vi "cubic and deadbands subvi.vi"(8 "Axis2":dbl, 9 "Axis1":dbl) -> (2 "Axis2":dbl, 3 "Axis1":dbl)   [LabVIEW 2017]
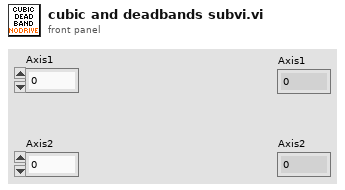
[diagram p1: front panel]
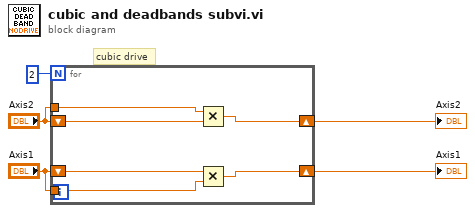
[diagram p0: block diagram]
diagram:
  # "cubic drive"
  n1 = for {
    N: 2 -> [_]
    shift-right: [w6] -> w3
    shift-left: "Axis1" -> [w11]
    shift-right: [w7] -> w4
    shift-left: "Axis2" -> [w9]
    tunnel: "Axis1" -> [w10]
    tunnel: "Axis2" -> [w8]
    n2 = Multiply(x=w8, y=w9) -> (x*y=w7:dbl)
    n3 = Multiply(x=w11, y=w10) -> (x*y=w6:dbl)
  }
  "Axis1" <- w3
  "Axis2" <- w4
